vi "Create User Buffer.vi"(0 "VISA resource name":refnum<visa-resource-name>, 5 "Buffer Name":string, 7 "Buffer Size":i32 min=10 step=1, 11 "error in (no error)":errorcluster) -> (4 "VISA resource name out":refnum<visa-resource-name>, 15 "error out":errorcluster)   [LabVIEW 2009, in "Keithley DMM7510.lvlib"]
doc: "This VI creates a user-defined reading buffer.\nYou cannot assign user-defined reading buffers the same name as an existing buffer, including the default buffers (defbuffer1 and defbuffer2)."
uses:
  Keithley DMM7510.lvlib
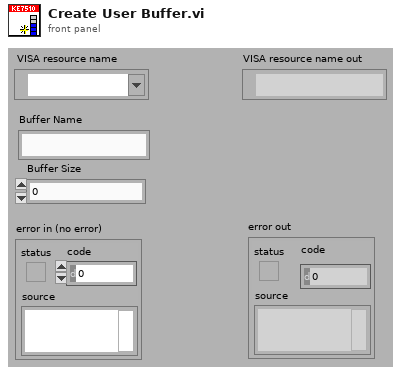
[diagram p1: front panel]
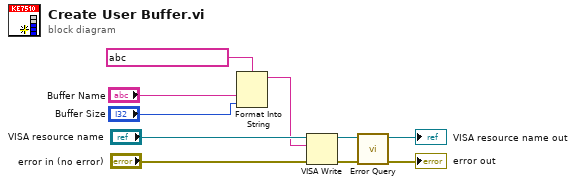
[diagram p0: block diagram]
diagram:
  n1 = Format Into String(format string=string ? ("Read Measurement"), "Buffer Name", "Buffer Size") -> (resulting string=w1:string)  [unwired: 2 in, 1 out]
  n2 = VISA Write(VISA resource name="VISA resource name", write buffer=w1, error in (no error)="error in (no error)") -> (VISA resource name out=w6:refnum<visa-resource-name>, error out=w5:errorcluster)  [unwired: 1 out]
  n3 = call "Error Query.vi"("error in (no error)"=w5, "VISA resource name"=w6) -> ("error out"=→"error out":errorcluster, "VISA resource name out"=→"VISA resource name out":refnum<visa-resource-name>)  [unwired: 8 out]
